vi "Insert Data into Controller CVT.vi"(6 "Update MSG":string, 7 "Group":string, 8 "error in":errorcluster, 9 "Data":variant, 10 "tag":string, 11 "Actor in":refnum<class "Actor.lvclass">) -> (0 "error out":errorcluster, 3 "Actor Out":refnum<class "Actor.lvclass">)   [LabVIEW 2017, in "Controller.lvlib" / "gController.lvclass"]
uses:
  gController.lvclass
  <vilib>/ActorFramework/Actor/Actor.lvclass
  <vilib>/MSR Consulting, LLC/General Reuse/SuperActor/SuperActor.lvclass
  C:/Program Files (x86)/National Instruments/LabVIEW 2017/vi.lib/ActorFramework/Actor/Actor.lvclass
  <vilib>/MSR Consulting, LLC/General Reuse/SuperActor/SuperActor.lvclass/SuperActor.ctl
  <vilib>/MSR Consulting, LLC/General Reuse/SuperActor/Read CVT Session.vi
  <vilib>/MSR Consulting, LLC/General Reuse/SuperActor/Read Log Session.vi
  <vilib>/MSR Consulting, LLC/General Reuse/Session APIs/_Session Fwk/Session - Root.lvclass
  <vilib>/MSR Consulting, LLC/General Reuse/Session APIs/CVT/CVT.lvclass
  <vilib>/MSR Consulting, LLC/General Reuse/Session APIs/Session Log/System Log.lvclass
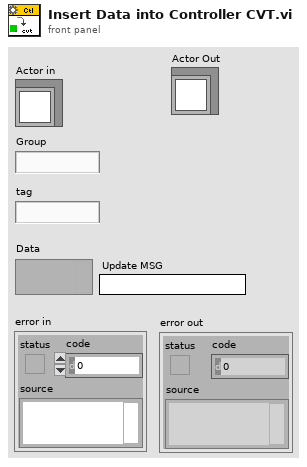
[diagram p1: front panel]
types:
  T1 = typedef "Session - Root.lvclass/Session Handle.ctl" = refnum<data-value>
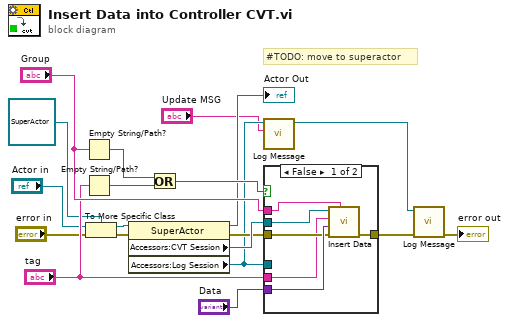
[diagram p0: block diagram]
diagram:
  # "#TODO: move to superactor"
  n1 = Empty String/Path?(string/path="Group") -> (empty?=w16:bool)
  n2 = Empty String/Path?(string/path="tag") -> (empty?=w15:bool)
  n3 = To More Specific Class(target class=refnum<class "SuperActor.lvclass"> refnum ("SuperActor.lvlib:SuperActor"), reference="Actor in", error in="error in") -> (specific class reference=w9:refnum<class "SuperActor.lvclass">, error out=w6:errorcluster)
  n4 = property class="SuperActor"(reference=w9, error in=w6) -> (reference out=→"Actor Out":refnum<class "SuperActor.lvclass">, error out=w17:errorcluster, "Accessors:CVT Session"=w19:T1, "Accessors:Log Session"=w4:T1)
  n5 = Or(x=w16, y=w15) -> (x .or. y?=w12:bool)
  n6 = call <vilib>:"Log Message.vi"("MSG In"="Update MSG", "session in"=w4) -> ("session out"=w3:T1)  [unwired: 8 in, 1 out]
  n7 = case shown="False" w12 {
    tunnel: w19 -> [w25 _]
    tunnel: "Data" -> [w24 _]
    tunnel: w17 -> [w23 w26]
    tunnel: [w22 w26] -> w5
    tunnel: "Group" -> [w21 _]
    tunnel: "tag" -> [w20 _]
    tunnel: w4 -> [_ _]
    frame False {
      n8 = call <vilib>:"Insert Data.vi"("Group"=w21, "error in"=w23, "Data"=w24, "tag"=w20, "CVT Session In"=w25) -> ("error out"=w22:errorcluster)  [unwired: 5 in, 1 out]
    }
    frame True {
    }
  }
  n9 = call <vilib>:"Log Message.vi"("error in"=w5, "session in"=w3) -> ("error out"=→"error out":errorcluster)  [unwired: 8 in, 1 out]
